vi "Save Calibration.vi"(0 "VISA resource name":refnum<visa-resource-name>, 11 "error in (no error)":errorcluster) -> (4 "VISA resource name out":refnum<visa-resource-name>, 15 "error out":errorcluster)   [LabVIEW 2020, in "NH Research Regenerative Test Series.lvlib"]
doc: "This command saves all the calibration factors in RAM to flash."
uses:
  NH Research Regenerative Test Series.lvlib
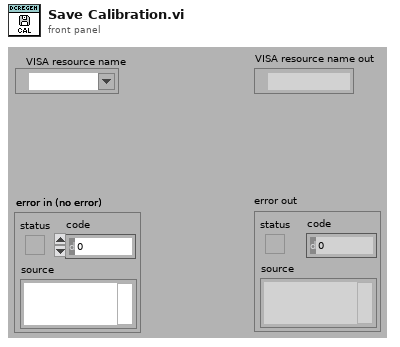
[diagram p1: front panel]
types:
  T1 = typedef "LVDateTimeRec.ctl" = cluster{"fractional second":dbl, "second":i32, "minute":i32, "hour":i32, "day of month":i32, "month":i32, "year":i32, "day of week":i32, "day of year":i32, "DST":i32}
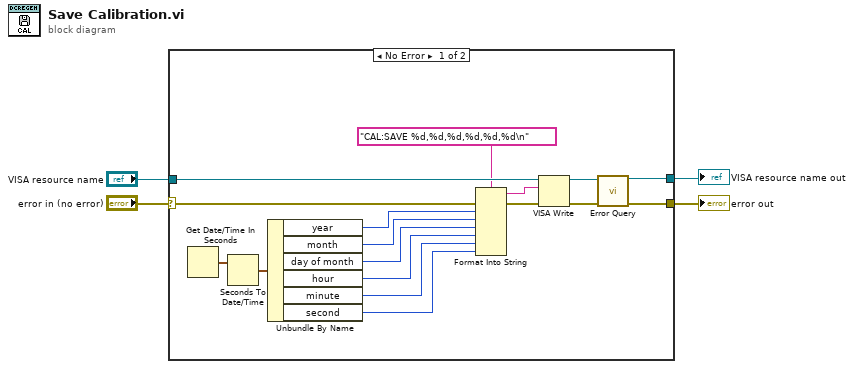
[diagram p0: block diagram]
diagram:
  n1 = case shown="No Error" "error in (no error)" {
    selector: "error in (no error)" -> [w18 w23]
    tunnel: [w5 w23] -> w3
    tunnel: [w20 w22] -> w1
    tunnel: "VISA resource name" -> [w21 w22]
    frame No Error {
      n2 = Get Date/Time In Seconds() -> (seconds since 1Jan1904=w8:timestamp)
      n3 = Seconds To Date/Time(time stamp (now)=w8) -> (date time rec=w16:T1)  [unwired: 1 in]
      n4 = Unbundle By Name(w16) -> ("year"=w15:i32, "month"=w14:i32, "day of month"=w13:i32, "hour"=w12:i32, "minute"=w11:i32, "second"=w10:i32)
      n5 = Format Into String(format string="CAL:SAVE %d,%d,%d,%d,%d,%d\n", error in=w18, w15, w14, w13, w12, w11, w10) -> (resulting string=w9:string, error out=w17:errorcluster)  [unwired: 1 in]
      n6 = VISA Write(VISA resource name=w21, write buffer=w9, error in (no error)=w17) -> (VISA resource name out=w6:refnum<visa-resource-name>, error out=w7:errorcluster)  [unwired: 1 out]
      n7 = call "Error Query.vi"("VISA resource name"=w6, "error in (no error)"=w7) -> ("VISA resource name out"=w20:refnum<visa-resource-name>, "error out"=w5:errorcluster)  [unwired: 10 in, 2 out]
    }
    frame Error {
    }
  }
  "error out" <- w3
  "VISA resource name out" <- w1
